vi "test Get Attribute as JSON with Sub Object.vi"(11 "Test Case In":refnum<class "Test Config From Excel Table.lvclass">) -> (0 "error out":errorcluster, 3 "Test Case Out":refnum<class "Test Config From Excel Table.lvclass">)   [LabVIEW 2020, in "Test Config From Excel Table.lvclass"]
uses:
  Test Config From Excel Table.lvclass
  C:/Program Files/National Instruments/LabVIEW 2025/vi.lib/Astemes/LUnit/Test Case.lvclass
  Source/Config from Excel Table/Config from Excel Table.lvclass
  <vilib>/Astemes/LUnit/Test Case.lvclass/Test Case.ctl
  Test Config From Excel Table.lvclass/Test Config From Excel Table.ctl
  <vilib>/JDP Science/JSONtext/JSONtext.lvlib
  <vilib>/Astemes/LUnit/Test Case.lvclass
  <vilib>/Peter/Open Xml/Source/Open Xml.lvlib
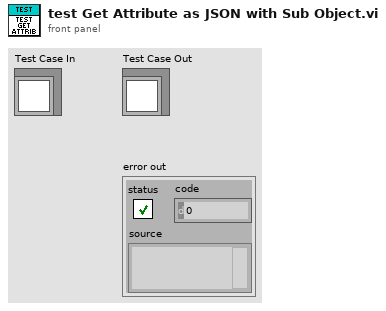
[diagram p1: front panel]
types:
  T1 = cluster{"Sheet Name":string, "Name":string, "Display Name":string, "Range or Cell Address":string}
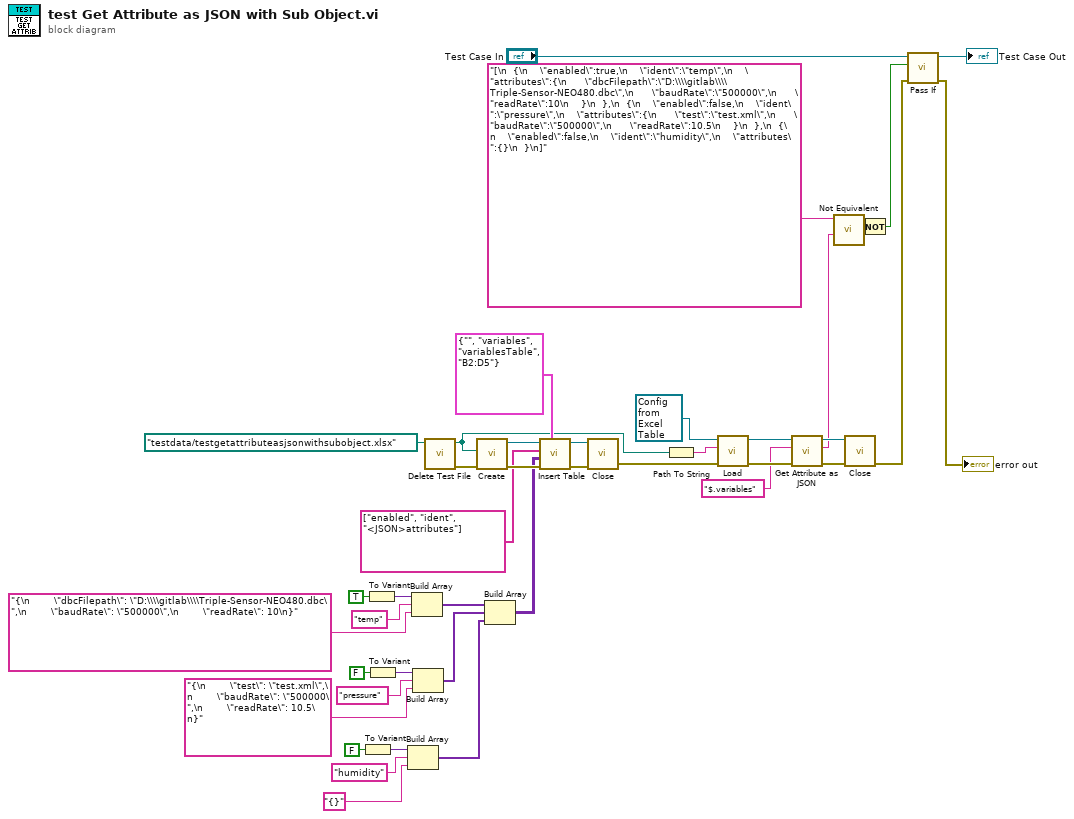
[diagram p0: block diagram]
diagram:
  n1 = To Variant(anything=FALSE) -> (Variant=w15:variant)
  n2 = To Variant(anything=TRUE) -> (Variant=w23:variant)
  n3 = To Variant(anything=FALSE) -> (Variant=w18:variant)
  n4 = Build Array(w15, "humidity", "{}") -> (w11:variant[])
  n5 = Build Array(w23, "temp", "{\n        \"dbcFilepath\": \"D:\\\\gitlab\\\\Triple-Sensor-NEO480.dbc\",\n        \"baudRate\": \"500000\",\n        \"readRate\": 10\n}") -> (w20:variant[])
  n6 = Build Array(w18, "pressure", "{\n        \"test\": \"test.xml\",\n        \"baudRate\": \"500000\",\n        \"readRate\": 10.5\n}") -> (w12:variant[])
  n7 = call "Delete Test File.vi"("name or relative path"=path "testdata/testgetattributeasjsonwithsubobject.xlsx") -> ("error out"=w28:errorcluster, "deleted path"=w2:path)  [unwired: 9 in]
  n8 = call <vilib>:"Create.vi"("error in"=w28, "Path"=w2) -> ("error out"=w27:errorcluster, "SpreadsheetDoc"=w9:refnum<k24>)  [unwired: 8 in]
  n9 = Build Array(w20, w12, w11) -> (w10:variant[][])
  n10 = call <vilib>:"Insert Table.vi"("Location"=T1 {"Sheet Name"="", "Name"="variables", "Display Name"="variablesTable", "Range or Cell Address"="B2:D5"}, "error in"=w27, "Cell Values"=w10, "Header Names"=string[] ["enabled", "ident", "<JSON>attributes"], "SpreadsheetDoc in"=w9) -> ("error out"=w8:errorcluster, "SpreadsheetDoc out"=w7:refnum<k24>)  [unwired: 5 in]
  n11 = call <vilib>:"Close.vi"("error in"=w8, "SpreadsheetDoc"=w7) -> ("error out"=w6:errorcluster)  [unwired: 9 in]
  n12 = Path To String(path=w2) -> (string=w38:string)
  n13 = call-dynamic "Load.vi"("error in"=w6, "Source"=w38, "Config from Excel Table in"=refnum<class "Config from Excel Table.lvclass"> refnum ("Config from EXCEL Table.lvclass")) -> ("error out"=w35:errorcluster, "Config from Excel Table out"=w36:refnum<class "Config from Excel Table.lvclass">)  [unwired: 7 in]
  n14 = call-dynamic "Get Attribute as JSON.vi"("error in"=w35, "Attribute"="$.variables", "Config from Excel Table in"=w36) -> ("error out"=w33:errorcluster, "<JSON>"=w29:string, "Config from Excel Table out"=w32:refnum<class "Config from Excel Table.lvclass">)  [unwired: 6 in]
  n15 = call <vilib>:"Not Equivalent.vi"("Other JSON"=w29, "JSON"="[\n  {\n    \"enabled\":true,\n    \"ident\":\"temp\",\n    \"attributes\":{\n      \"dbcFilepath\":\"D:\\\\gitlab\\\\Triple-Sensor-NEO480.dbc\",\n      \"baudRate\":\"500000\",\n      \"readRate\":10\n    }\n  },\n  {\n    \"enabled\":false,\n    \"ident\":\"pressure\",\n    \"attributes\":{\n      \"test\":\"test.xml\",\n      \"baudRate\":\"500000\",\n      \"readRate\":10.5\n    }\n  },\n  {\n    \"enabled\":false,\n    \"ident\":\"humidity\",\n    \"attributes\":{}\n  }\n]" ("<JSON>")) -> ("Not Equivalent"=w31:bool)  [unwired: 8 in]
  n16 = call-dynamic <vilib>:"Close.vi"("error in"=w33, "Config from Excel Table in"=w32) -> ("error out"=w37:errorcluster)  [unwired: 8 in, 1 out]
  n17 = Not(x=w31) -> (.not. x?=w30:bool)
  n18 = call <vilib>:"Pass If.vi"("error in (no error)"=w37, "Pass?"=w30, "LUnit Test Case In"="Test Case In") -> ("error out"=→"error out":errorcluster, "LUnit Test Case Out"=→"Test Case Out":refnum<class "Test Config From Excel Table.lvclass">)  [unwired: 7 in]
